vi "Set MLJ Stage Enabled.vi"(8 "error in (no error)":errorcluster, 9 "Enable/Disable":bool, 10 "Cluster in":T1, 11 "MLJ Reference In":refnum<k24>) -> (0 "error out":errorcluster, 2 "Cluster out":T1, 3 "MLJ Reference Out":refnum<k24>)   [LabVIEW 2017]
uses:
  Controls/Translation Stage Cluster.ctl
  General/Controls/Translation Stage Types.ctl
  C:/Users/OCT/Documents/SD-OCT-master/SD-OCT-master/Software/Thorlabs.MotionControl.Controls.dll
  Thorlabs.MotionControl.Controls.dll
  C:/Users/OCT/Documents/SD-OCT-master/SD-OCT-master/Software/Thorlabs.MotionControl.IntegratedStepperMotorsCLI.dll
  Thorlabs.MotionControl.IntegratedStepperMotorsCLI.dll
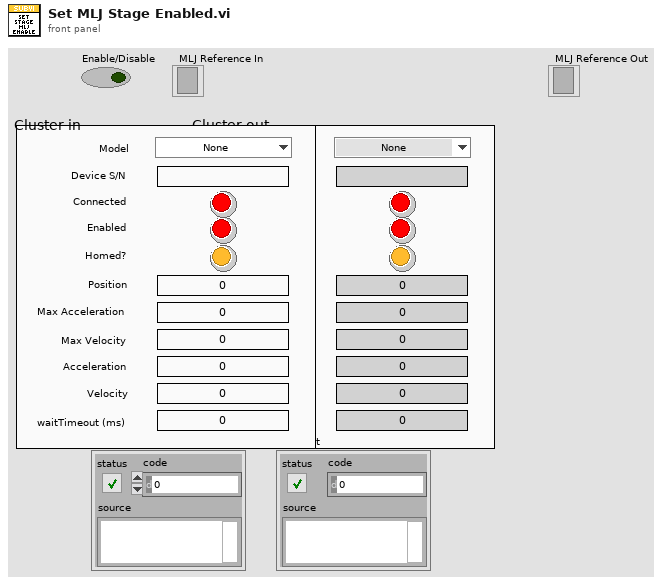
[diagram p1: front panel]
types:
  T1 = typedef "Translation Stage Cluster.ctl" = cluster{"Position":dbl, "Is.Enabled?":bool, "Is.Connected?":bool, "Device SN":string, "AccelerationMaximum":dbl, "VelocityMaximum":dbl, "Acceleration":dbl, "Velocity":dbl, "waitTimeout (ms)":i32, "Model":T2, "Is.Homed?":bool}
  T2 = typedef "Translation Stage Types.ctl" = enum16{"None", "Thorlabs LTS", "Thorlabs MLJ"}
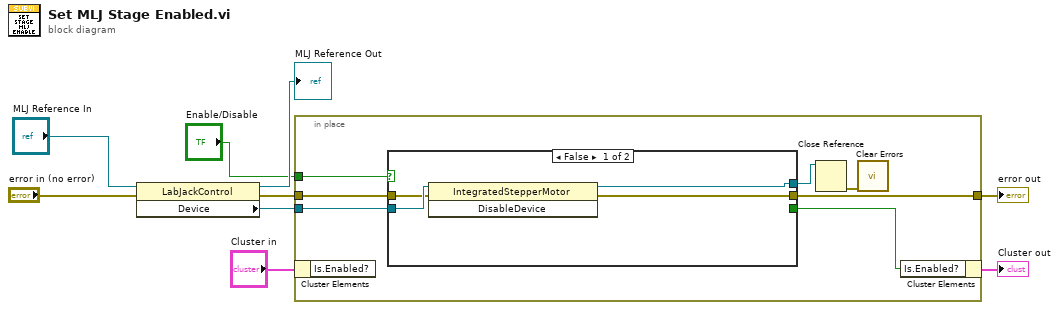
[diagram p0: block diagram]
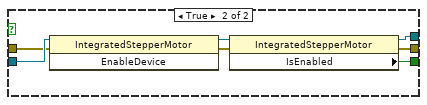
[diagram p2: hidden frame]
diagram:
  n1 = property class="LabJackControl"(reference="MLJ Reference In", error in="error in (no error)") -> (reference out=→"MLJ Reference Out":refnum<k24>, error out=w7:errorcluster, "Device"=w3:refnum<k24>)
  n2 = in-place {
    in-place-border: w3 -> [w16]
    in-place-border: w7 -> [w15]
    in-place-border: [w14] -> w5
    in-place-border: "Enable/Disable" -> [w10]
    n3 = in-place-cluster #1("Cluster in") -> ()  [unwired: 1 out]
    n4 = case shown="False" w10 {
      tunnel: w16 -> [w20 w27]
      tunnel: w15 -> [w19 w26]
      tunnel: [w18 w24] -> w14
      tunnel: [w17 w22] -> w12
      tunnel: [_ w21] -> w11
      frame False {
        n5 = invoke class="IntegratedStepperMotor" method="DisableDevice"(reference=w20, error in=w19) -> (reference out=w17:refnum<k24>, error out=w18:errorcluster)  [unwired: 1 in, 1 out]
      }
      frame True {
        n6 = invoke class="IntegratedStepperMotor" method="EnableDevice"(reference=w27, error in=w26) -> (reference out=w23:refnum<k24>, error out=w25:errorcluster)  [unwired: 1 in, 1 out]
        n7 = property class="IntegratedStepperMotor"(reference=w23, error in=w25) -> (reference out=w22:refnum<k24>, error out=w24:errorcluster, "IsEnabled"=w21:bool)
      }
    }
    n8 = Close Reference(reference=w12) -> (error out=w13:errorcluster)  [unwired: 1 in]
    n9 = call <vilib>:"Clear Errors.vi"("error in (no error)"=w13) -> ()  [unwired: 5 in, 2 out]
    n10 = in-place-cluster #1("Is.Enabled?"=w11) -> (→"Cluster out":T1)
  }
  "error out" <- w5
